vi "test_Analog PWM In.vi"(8 "error in (no error)":errorcluster, 11 "TestCase in":refnum<class "FPGA Addon Speciality IO Tests.lvclass">) -> (0 "error out":errorcluster, 3 "TestCase out":refnum<class "FPGA Addon Speciality IO Tests.lvclass">)   [LabVIEW 2018, in "FPGA Addon Speciality IO Tests.lvclass"]
uses:
  FPGA Addon Speciality IO Tests.lvclass
  D:/GitBranches/niveristand-custom-device-testing-tools/VeriStandTestCase/VeriStandTestCase.lvclass
  types/Channel Config.ctl
  <vilib>/addons/_JKI Toolkits/VI Tester/TestCase.llb/TestCase.lvclass
  FPGA Addon Test Class/FPGA Addon Test Class.lvclass
  C:/Program Files (x86)/National Instruments/LabVIEW 2018/vi.lib/addons/_JKI Toolkits/VI Tester/TestCase.llb/TestCase.lvclass
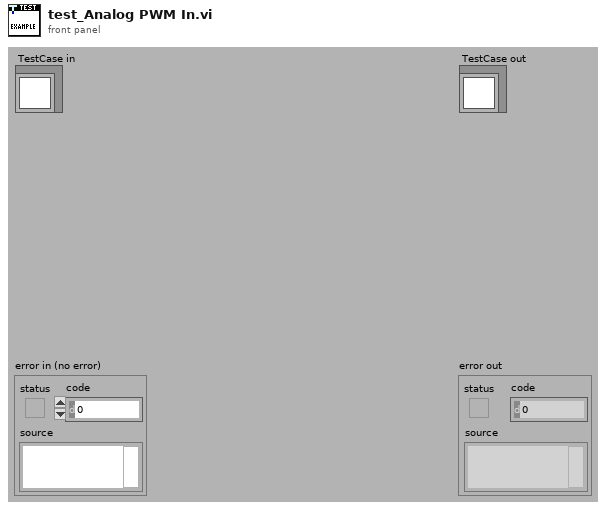
[diagram p1: front panel]
types:
  T1 = typedef "FPGA Addon Speciality IO Tests.lvclass/Channel Config.ctl" = cluster{"Scalar Output":string, "Scalar Input":string, "milliseconds to wait":u32, "Value":dbl}
  T2 = typedef "NI_VS Workspace ExecutionAPI.lvlib/WorkspaceAPI.ctl" = refnum<k24>
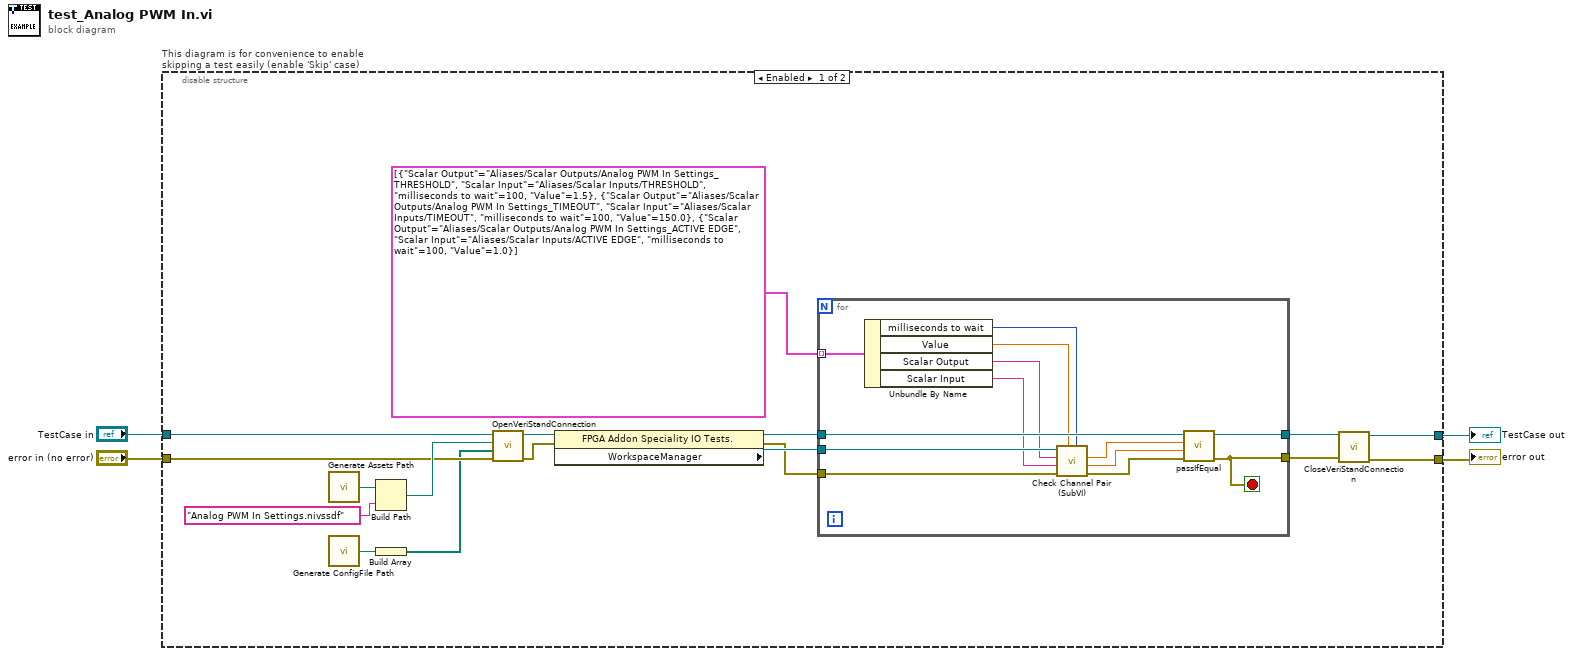
[diagram p0: block diagram]
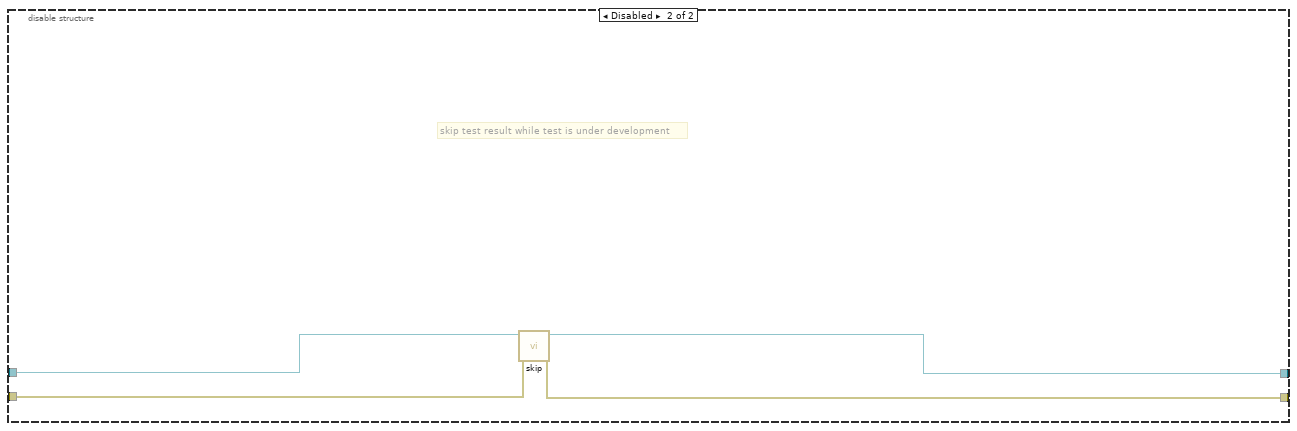
[diagram p2: hidden frame]
diagram:
  n1 = disable-structure "This diagram is for convenience to enable skipping a test easily (enable 'Skip' case)" shown="Enabled" {
    disable-tunnel: "TestCase in" -> [w14 w38]
    disable-tunnel: [w9 w36] -> w1
    disable-tunnel: [w10 w37] -> w3
    disable-tunnel: "error in (no error)" -> [w12 w35]
    frame Enabled {
      n2 = call "Generate Assets Path.vi"() -> ("Assets path"=w16:path)
      n3 = call "Generate ConfigFile Path.vi"() -> ("ConfigFile path"=w8:path)
      n4 = Build Path(base path=w16, name or relative path="Analog PWM In Settings.nivssdf") -> (appended path=w13:path)
      n5 = Build Array(w8) -> (w11:path[])
      n6 = call-dynamic "OpenVeriStandConnection.vi"("error in (no error)"=w12, "overrides files"=w11, "System Definition File"=w13, "VeriStand Test Case in"=w14) -> ("error out"=w21:errorcluster, "VeriStand Test Case out"=w20:refnum<class "FPGA Addon Speciality IO Tests.lvclass">)  [unwired: 5 in, 1 out]
      n7 = property class="FPGA Addon Speciality IO Tests."(reference=w20, error in=w21) -> (reference out=w19:refnum<class "FPGA Addon Speciality IO Tests.lvclass">, error out=w17:errorcluster, "WorkspaceManager"=w18:T2)
      n8 = for {
        tunnel: w19 -> [w34]
        tunnel: w18 -> [w33]
        tunnel: w17 -> [w31]
        tunnel: T1[] [{"Scalar Output"="Aliases/Scalar Outputs/Analog PWM In Settings_THRESHOLD", "Scalar Input"="Aliases/Scalar Inputs/THRESHOLD", "milliseconds to wait"=100, "Value"=1.5}, {"Scalar Output"="Aliases/Scalar Outputs/Analog PWM In Settings_TIMEOUT", "Scalar Input"="Aliases/Scalar Inputs/TIMEOUT", "milliseconds to wait"=100, "Value"=150.0}, {"Scalar Output"="Aliases/Scalar Outputs/Analog PWM In Settings_ACTIVE EDGE", "Scalar Input"="Aliases/Scalar Inputs/ACTIVE EDGE", "milliseconds to wait"=100, "Value"=1.0}] -> [w28] mode=indexing
        tunnel: [w23] -> w6
        tunnel: [w22] -> w5
        stop <- w23 stop-if-true
        n9 = Unbundle By Name(w28) -> ("milliseconds to wait"=w25:u32, "Value"=w24:dbl, "Scalar Output"=w27:string, "Scalar Input"=w26:string)
        n10 = call "Check Channel Pair (SubVI).vi"("milliseconds to wait"=w25, "Test Value"=w24, "error in (no error)"=w31, "Input Channel"=w26, "Output Channel"=w27, "WorkspaceManager in"=w33) -> ("error out"=w32:errorcluster, "InputChannel Value"=w29:dbl, "OutputChannel Value"=w30:dbl)  [unwired: 2 in, 1 out]
        n11 = call-dynamic "passIfEqual.vi"("error in (no error)"=w32, "y"=w29, "x"=w30, "TestCase in"=w34) -> ("error out"=w23:errorcluster, "TestCase out"=w22:refnum<class "FPGA Addon Speciality IO Tests.lvclass">)  [unwired: 6 in]
      }
      n12 = call-dynamic "CloseVeriStandConnection.vi"("error in (no error)"=w6, "VeriStand Test Case in"=w5) -> ("error out"=w10:errorcluster, "VeriStand Test Case out"=w9:refnum<class "FPGA Addon Speciality IO Tests.lvclass">)  [unwired: 8 in]
    }
    frame Disabled {
      # "skip test result while test is under development"
      n13 = call <vilib>:"skip.vi"("error in (no error)"=w35, "TestCase in"=w38) -> ("error out"=w37:errorcluster, "TestCase out"=w36:refnum<class "FPGA Addon Speciality IO Tests.lvclass">)  [unwired: 8 in]
    }
  }
  "error out" <- w3
  "TestCase out" <- w1
